vi "Connect.vi"(8 "error in (no error)":errorcluster, 11 "TCP Comm":T1) -> (0 "error out":errorcluster)   [LabVIEW 2020, in "TinyTCP.lvlib"]
uses:
  TinyTCP.lvlib
  Instance.ctl
  Ref Data.ctl
  State.ctl
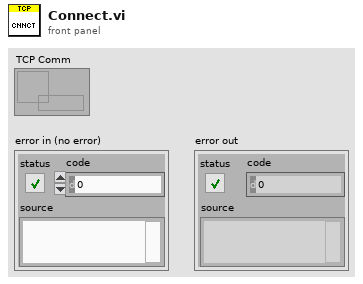
[diagram p1: front panel]
types:
  T1 = typedef "TinyTCP.lvlib/Instance.ctl" = refnum<data-value>
  T2 = typedef "TinyTCP.lvlib/Ref Data.ctl" = cluster{"TCP":refnum<k5>, "State":T3, "Server":bool, "Host":string, "Port":u16, "Listener":refnum<k5>, "Start":bool, "Disconnect":bool, "TCP Valid":bool, "TLS Enabled":bool, "Immutable TLS":refnum<k36>, "Certificate DN":string, "local-port":u16}
  T3 = typedef "TinyTCP.lvlib/State.ctl" = enum16{"Idle", "Starting", "Connecting", "Connected", "Disconnecting", "Stopped"}
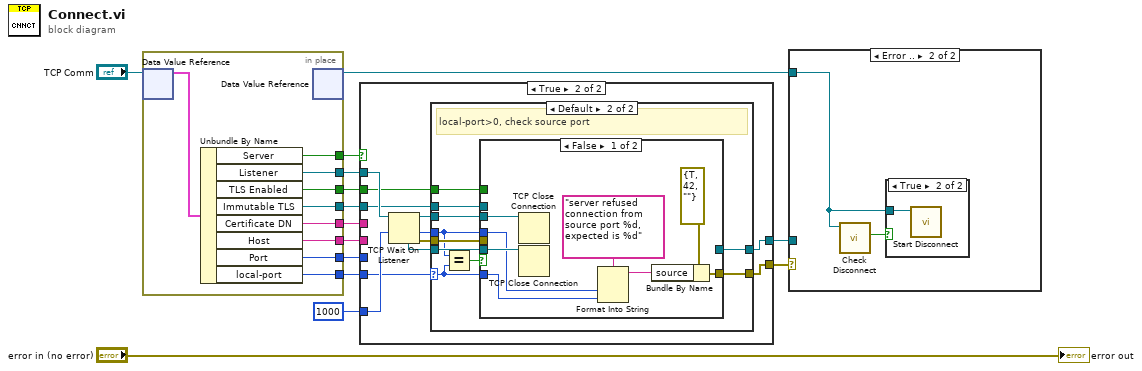
[diagram p0: block diagram]
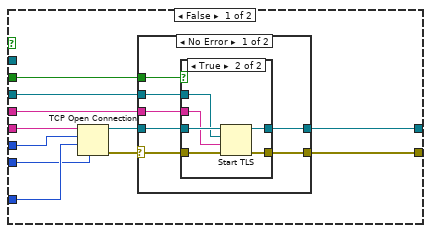
[diagram p2: hidden frame]
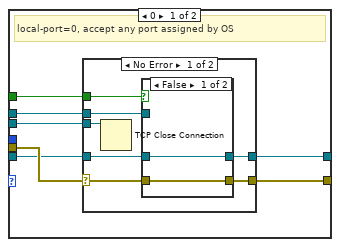
[diagram p5: hidden frame]
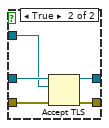
[diagram p6: hidden frame]
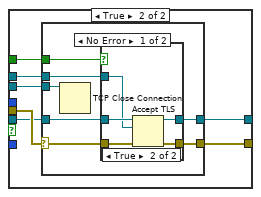
[diagram p8: hidden frame]
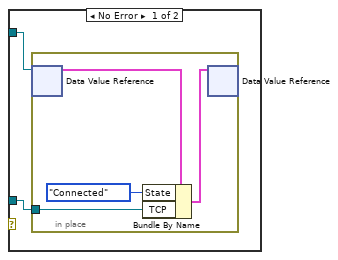
[diagram p11: hidden frame]
diagram:
  n1 = in-place {
    in-place-border: [w22] -> w12
    in-place-border: [w21] -> w13
    in-place-border: [w20] -> w6
    in-place-border: [w19] -> w5
    in-place-border: [w18] -> w4
    in-place-border: [w17] -> w3
    in-place-border: [w16] -> w2
    in-place-border: [w15] -> w1
    n2 = in-place-dvr #1("TCP Comm") -> (w23:T2)  [unwired: 1 out]
    n3 = Unbundle By Name(w23) -> ("Server"=w17:bool, "Listener"=w16:refnum<k5>, "TLS Enabled"=w19:bool, "Immutable TLS"=w20:refnum<k36>, "Certificate DN"=w18:string, "Host"=w22:string, "Port"=w21:u16, "local-port"=w15:u16)
    n4 = in-place-dvr #1() -> (w8:T1)  [unwired: 1 in, 1 out]
  }
  n5 = case shown="True" w3 {
    tunnel: w13 -> [w33 _]
    tunnel: w12 -> [w34 _]
    tunnel: [w27 w54] -> w10
    tunnel: [w25 w55] -> w9
    tunnel: 1000 ("timeout ms (wait forever: -1)") -> [w32 w61]
    tunnel: w6 -> [w28 w58]
    tunnel: w5 -> [w29 w59]
    tunnel: w4 -> [w26 _]
    tunnel: w2 -> [_ w60]
    tunnel: w1 -> [w24 w52]
    frame False {
      n6 = TCP Open Connection(address=w34, remote port or service name=w33, timeout ms (60000)=w32, local port=w24) -> (connection ID=w30:refnum<k5>, error out=w31:errorcluster)  [unwired: 1 in]
      n7 = case shown="No Error" w31 {
        selector: w31 -> [w41 w50]
        tunnel: w30 -> [w40 _]
        tunnel: w29 -> [w38 _]
        tunnel: w28 -> [w37 _]
        tunnel: [w35 w50] -> w27
        tunnel: w26 -> [w39 _]
        tunnel: [w36 _] -> w25
        frame No Error {
          n8 = case shown="True" w38 {
            tunnel: w41 -> [w42 w49]
            tunnel: w40 -> [w43 w48]
            tunnel: w39 -> [_ w47]
            tunnel: w37 -> [_ w46]
            tunnel: [w43 w45] -> w36
            tunnel: [w42 w44] -> w35
            frame False {
            }
            frame True {
              n9 = Start TLS(8:w49, 9:w47, 10:w46, 11:w48) -> (0:w44:errorcluster, 3:w45:refnum<k5>)  [unwired: 2 in, 1 out]
            }
          }
        }
        frame Error {
        }
      }
    }
    frame True {
      n10 = TCP Wait On Listener(9:w61, 11:w60) -> (0:w57:errorcluster, 1:w51:u16, 3:w53:refnum<k5>, 4:w56:refnum<k5>)  [unwired: 2 in, 1 out]
      n11 = case shown="Default" w52 {
        selector: w52 -> [_ w84]
        tunnel: w59 -> [w68 w93]
        tunnel: w58 -> [w67 w92]
        tunnel: w57 -> [w66 w91]
        tunnel: w56 -> [w65 w90]
        tunnel: [w64 w89] -> w55
        tunnel: [w63 w88] -> w54
        tunnel: w53 -> [w62 w87]
        tunnel: w51 -> [_ w85]
        frame 0 {
          # "local-port=0, accept any port assigned by OS"
          n12 = case shown="No Error" w66 {
            selector: w66 -> [w75 w83]
            tunnel: w65 -> [w74 _]
            tunnel: w68 -> [w73 _]
            tunnel: w67 -> [w72 _]
            tunnel: [w70 w83] -> w63
            tunnel: [w71 _] -> w64
            tunnel: w62 -> [w69 _]
            frame No Error {
              n13 = TCP Close Connection(connection ID=w69) -> ()  [unwired: 2 in, 2 out]
              n14 = case shown="False" w73 {
                tunnel: w75 -> [w76 w82]
                tunnel: w74 -> [w77 w81]
                tunnel: w72 -> [_ w80]
                tunnel: [w77 w79] -> w71
                tunnel: [w76 w78] -> w70
                frame False {
                }
                frame True {
                  n15 = Accept TLS(8:w82, 10:w80, 11:w81) -> (0:w78:errorcluster, 3:w79:refnum<k5>)  [unwired: 1 in, 1 out]
                }
              }
            }
            frame Error {
            }
          }
        }
        frame Default {
          # "local-port>0, check source port"
          n16 = Equal?(x=w85, y=w84) -> (x = y?=w86:bool)
          n17 = case shown="False" w86 {
            tunnel: w93 -> [_ w108]
            tunnel: w92 -> [_ w107]
            tunnel: w91 -> [_ w106]
            tunnel: w90 -> [w100 w105]
            tunnel: [_ w104] -> w89
            tunnel: [w98 w103] -> w88
            tunnel: w87 -> [w101 w102]
            tunnel: w85 -> [w95 _]
            tunnel: w84 -> [w94 _]
            frame False {
              n18 = TCP Close Connection(connection ID=w101) -> ()  [unwired: 2 in, 2 out]
              n19 = TCP Close Connection(connection ID=w100) -> ()  [unwired: 2 in, 2 out]
              n20 = Format Into String(format string="server refused connection from source port %d, expected is %d" ("source"), w95, w94) -> (resulting string=w97:string)  [unwired: 2 in, 1 out]
              n21 = Bundle By Name(cluster=errorcluster {"status"=TRUE, "code"=42, "source"=""} ("error IO"), "source"=w97) -> (w98:errorcluster)
            }
            frame True {
              n22 = case shown="No Error" w106 {
                selector: w106 -> [w115 w123]
                tunnel: w105 -> [w114 _]
                tunnel: w108 -> [w113 _]
                tunnel: w107 -> [w112 _]
                tunnel: [w110 w123] -> w103
                tunnel: [w111 _] -> w104
                tunnel: w102 -> [w109 _]
                frame No Error {
                  n23 = TCP Close Connection(connection ID=w109) -> ()  [unwired: 2 in, 2 out]
                  n24 = case shown="True" w113 {
                    tunnel: w115 -> [w116 w122]
                    tunnel: w114 -> [w117 w121]
                    tunnel: w112 -> [_ w120]
                    tunnel: [w117 w119] -> w111
                    tunnel: [w116 w118] -> w110
                    frame False {
                    }
                    frame True {
                      n25 = Accept TLS(8:w122, 10:w120, 11:w121) -> (0:w118:errorcluster, 3:w119:refnum<k5>)  [unwired: 1 in, 1 out]
                    }
                  }
                }
                frame Error {
                }
              }
            }
          }
        }
      }
    }
  }
  n26 = case shown="Error .." w10 {
    tunnel: w9 -> [w124 _]
    tunnel: w8 -> [w125 w130]
    frame No Error {
      n27 = in-place {
        in-place-border: w124 -> [w127]
        n28 = in-place-dvr #2(w125) -> (w129:T2)  [unwired: 1 out]
        n29 = Bundle By Name(cluster=w129, "State"=State."Connected", "TCP"=w127) -> (w128:T2)
        n30 = in-place-dvr #2(w128) -> ()  [unwired: 2 out]
      }
    }
    frame Error {
      n31 = call "Check Disconnect.vi"("TCP Comm"=w130) -> ("Disconnecting?"=w131:bool)  [unwired: 9 in, 1 out]
      n32 = case shown="True" w131 {
        tunnel: w130 -> [_ w132]
        frame False {
        }
        frame True {
          n33 = call "Start Disconnect.vi"("TCP Comm"=w132) -> ()  [unwired: 10 in, 1 out]
        }
      }
    }
  }
  "error out" <- "error in (no error)"
